vi "Find System Folder.vi"(1 "Application Name":string="Unknown", 5 "error in (no error)":errorcluster, 6 "system directory type":T1 items=["User Home"=0, "User Desktop"=1, "User Documents"=2, "User Application Data"=3, "User Preferences"=4, "User Temporary"=5, "Public Documents"=6, "Public Application Data"=7, "Public Preferences"=8, "Public Cache"=13, "System Core Libraries"=9, "System Installed Libraries"=10, "Application Files"=11, "Boot Volume Root"=12]) -> (15 "System Folder":path, 19 "error out":errorcluster)   [LabVIEW 2020, in "Generic Utilities.lvclass"]
uses:
  Generic Utilities.lvclass
  <vilib>/Utility/sysdir.llb/System Directory Type.ctl
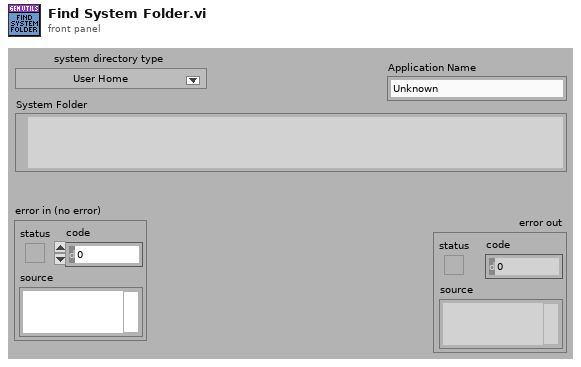
[diagram p1: front panel]
types:
  T1 = typedef "System Directory Type.ctl" = i32
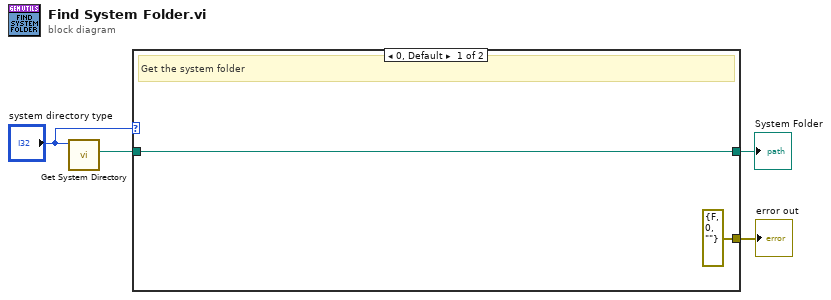
[diagram p0: block diagram]
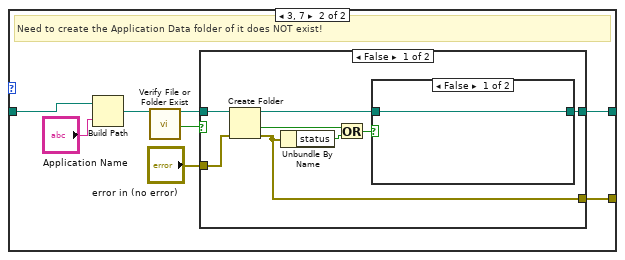
[diagram p2: hidden frame]
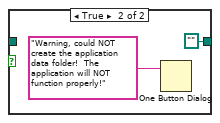
[diagram p3: hidden frame]
diagram:
  n1 = call <vilib>:"Get System Directory.vi"("system directory type"="system directory type") -> ("system directory"=w3:path)  [unwired: 10 in]
  n2 = case shown="0, Default" "system directory type" {
    tunnel: [errorcluster {"status"=FALSE, "code"=0, "source"=""} ("error in (no error)") w14] -> w4
    tunnel: w3 -> [w6 w12]
    tunnel: [w6 w11] -> w2
    frame 0, Default {
      # "Get the system folder"
    }
    frame 3, 7 {
      # "Need to create the Application Data folder of it does NOT exist!"
      n3 = Build Path(base path=w12, name or relative path="Application Name") -> (appended path=w9:path)
      n4 = call "Verify File or Folder Exist.vi"("path"=w9) -> ("dup path"=w8:path, "file or folder exists?"=w7:bool)  [unwired: 16 in, 1 out]
      n5 = case shown="False" w7 {
        tunnel: w8 -> [w22 w27]
        tunnel: [w18 w27] -> w11
        tunnel: "error in (no error)" -> [w16 w26]
        tunnel: [w15 w26] -> w14
        frame False {
          n6 = Create Folder(path (use dialog)=w22, error in=w16) -> (created path=w17:path, cancelled=w21:bool, error out=w15:errorcluster)  [unwired: 1 in]
          n7 = Unbundle By Name(w15) -> ("status"=w20:bool)
          n8 = Or(x=w21, y=w20) -> (x .or. y?=w19:bool)
          n9 = case shown="False" w19 {
            tunnel: [w23 path ""] -> w18
            tunnel: w17 -> [w23 _]
            frame False {
            }
            frame True {
              n10 = One Button Dialog(message="Warning, could NOT create the application data folder!  The application will NOT function properly!") -> ()  [unwired: 1 in, 1 out]
            }
          }
        }
        frame True {
        }
      }
    }
  }
  "System Folder" <- w2
  "error out" <- w4
